vi "Add FPGA Build Specs.vi"(10 "build spec details":T1, 11 "Number of Build Specs":i32) -> (3 "Added Build Specs":T2[](array[typedef]))   [LabVIEW 2013]
uses:
  <vilib>/rvi/CDR/niFpgaBuild_BuildSpecPath.ctl
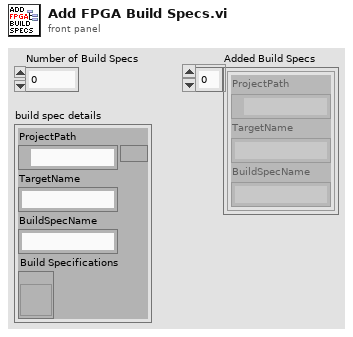
[diagram p1: front panel]
types:
  T1 = cluster{"ProjectPath":path, "TargetName":string, "BuildSpecName":string, "Build Specifications":refnum<vi>}
  T2 = typedef "niFpgaBuild_BuildSpecPath.ctl" = cluster{"ProjectPath":path, "TargetName":string, "BuildSpecName":string}
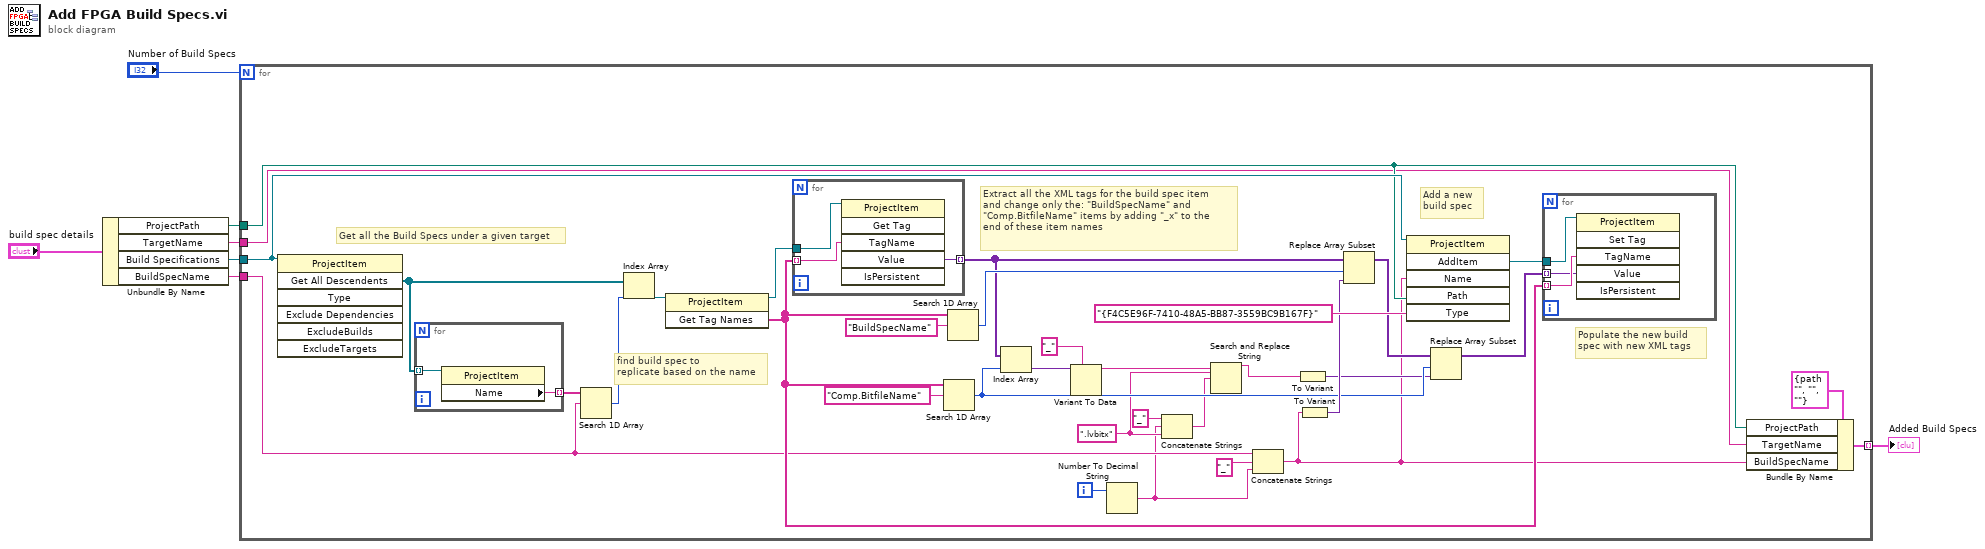
[diagram p0: block diagram]
diagram:
  n1 = Unbundle By Name("build spec details") -> ("ProjectPath"=w5:path, "TargetName"=w6:string, "Build Specifications"=w2:refnum<vi>, "BuildSpecName"=w4:string)
  n2 = for {
    N: "Number of Build Specs" -> [_]
    tunnel: w2 -> [w21]
    tunnel: w4 -> [w19]
    tunnel: w5 -> [w17]
    tunnel: w6 -> [w16]
    tunnel: [w14] -> w7 mode=indexing
    i -> [w25]
    w11 = ".lvbitx" ("search string")
    # "Extract all the XML tags for the build spec item\nand change only the: \"BuildSpecName\" and \n\"Comp.BitfileName\" items by adding \"_x\" to the\nend of these item names"
    # "Populate the new build \nspec with new XML tags"
    # "Add a new \nbuild spec"
    # "find build spec to \nreplicate based on the name"
    # "Get all the Build Specs under a given target"
    n3 = invoke class="ProjectItem" method="Get All Descendents"(reference=w21) -> ("All Descendents"=w22:refnum<vi>[])  [unwired: 6 in, 6 out]
    n4 = for {
      tunnel: [w43] -> w24 mode=indexing
      tunnel: w22 -> [w42] mode=indexing
      n5 = property class="ProjectItem"(reference=w42) -> ("Name"=w43:string)  [unwired: 1 in, 2 out]
    }
    n6 = Search 1D Array(1D array=w24, element=w19) -> (index of element=w23:i32)  [unwired: 1 in]
    n7 = Index Array(array=w22, index=w23) -> (element=w20:refnum<vi>)
    n8 = invoke class="ProjectItem" method="Get Tag Names"(reference=w20) -> (reference out=w39:refnum<vi>, "Get Tag Names"=w27:string[])  [unwired: 2 in, 1 out]
    n9 = for {
      tunnel: w39 -> [w46]
      tunnel: w27 -> [w45] mode=indexing
      tunnel: [w44] -> w30 mode=indexing
      n10 = invoke class="ProjectItem" method="Get Tag"(reference=w46, "TagName"=w45) -> ("Value"=w44:variant)  [unwired: 4 in, 5 out]
    }
    n11 = Search 1D Array(1D array=w27, element="Comp.BitfileName") -> (index of element=w34:i32)  [unwired: 1 in]
    n12 = Search 1D Array(1D array=w27, element="BuildSpecName") -> (index of element=w38:i32)  [unwired: 1 in]
    n13 = Index Array(array=w30, index=w34) -> (element=w28:variant)
    n14 = Variant To Data(type="_" ("string"), Variant=w28) -> (data=w12:string)  [unwired: 1 in, 1 out]
    n15 = Number To Decimal String(number=w25) -> (decimal integer string=w9:string)  [unwired: 1 in]
    n16 = Concatenate Strings("_" ("string"), w9, w11) -> (w10:string)
    n17 = Search and Replace String(input string=w12, search string=w11, replace string=w10) -> (result string=w8:string)  [unwired: 5 in, 3 out]
    n18 = Concatenate Strings(w19, "_" ("string"), w9) -> (w15:string)
    n19 = To Variant(anything=w8) -> (Variant=w33:variant)
    n20 = To Variant(anything=w15) -> (Variant=w37:variant)
    n21 = Replace Array Subset(array=w30, new element=w37, index=w38) -> (w32:variant[])
    n22 = invoke class="ProjectItem" method="AddItem"(reference=w21, "Name"=w15, "Path"=w17, "Type"="{F4C5E96F-7410-48A5-BB87-3559BC9B167F}") -> ("AddItem"=w40:refnum<vi>)  [unwired: 2 in, 5 out]
    n23 = Replace Array Subset(array=w32, new element=w33, index=w34) -> (w31:variant[])
    n24 = for {
      tunnel: w40 -> [w49]
      tunnel: w27 -> [w48] mode=indexing
      tunnel: w31 -> [w47] mode=indexing
      n25 = invoke class="ProjectItem" method="Set Tag"(reference=w49, "TagName"=w48, "Value"=w47) -> ()  [unwired: 3 in, 6 out]
    }
    n26 = Bundle By Name(cluster=T2 {"ProjectPath"=path "", "TargetName"="", "BuildSpecName"=""} ("build spec path"), "ProjectPath"=w17, "TargetName"=w16, "BuildSpecName"=w15) -> (w14:T2)
  }
  "Added Build Specs" <- w7
